vi "Actor.vi"(7 "ConcreteActor":refnum<class "ConcreteActor.lvclass">, 11 "ErrorQueue":refnum<queue>) -> (4 "Error":errorcluster, 5 "ConcreteActor":refnum<class "ConcreteActor.lvclass">)   [LabVIEW 2020, in "_Template.lvlib" / "ActorTemplate.lvlib" / "{{Name}}.lvlib" / "ConcreteActor.lvclass"]
uses:
  ConcreteActor.lvclass
  C:/jettl-harness/repos/jettl/src/jettl/jettl/Actor/Actor.lvclass
  ConcreteActor.lvclass/ConcreteActor.ctl
  jettl/jettl/jettl.lvlib
panel:
  # "This panel can be extended with controls and indicators, though do not modify the conn pane."
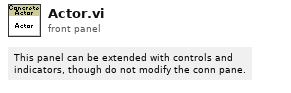
[diagram p1: front panel]
types:
  T1 = cluster{"EventRegistrationRef":refnum<event-registration>}
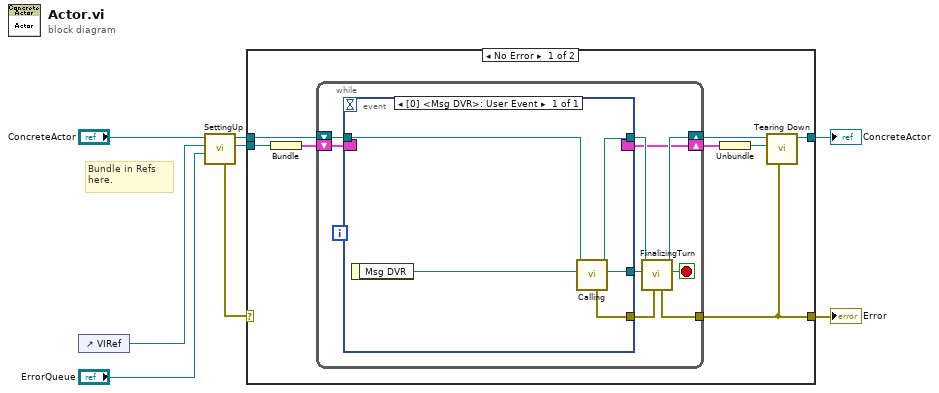
[diagram p0: block diagram]
diagram:
  # "Bundle in Refs here."
  n1 = control-ref of="VIRef"() -> (w3:refnum<vi>)
  n2 = call "SettingUp.vi"("ErrorQueue"="ErrorQueue", "VIRef"=w3, "Actor"="ConcreteActor") -> ("EventRegistrationRef"=w6:refnum<event-registration>, "Actor"=w4:refnum<class "ConcreteActor.lvclass">, "Error"=w1:errorcluster)  [unwired: 6 in]
  n3 = case shown="No Error" w1 {
    selector: w1 -> [_ w31]
    tunnel: [w11 w32] -> w8
    tunnel: w4 -> [w16 w32]
    tunnel: [w10 w31] -> w7
    tunnel: w6 -> [w15 _]
    frame No Error {
      n4 = Bundle("EventRegistrationRef"=w15) -> (w14:T1)  [unwired: 1 in]
      n5 = while {
        shift-right: [w18] -> w12
        shift-left: w16 -> [w25]
        tunnel: [w21] -> w10
        shift-right: [w17] -> w13
        shift-left: w14 -> [w23]
        stop <- w24 stop-if-true
        n6 = event shown="[0] <Msg DVR>: User Event" {
          selector: w23 -> [_]
          dyn-events: [_] -> w17
          timeout: _ -> [_]
          tunnel: w25 -> [w29]
          tunnel: [w28] -> w19
          tunnel: [w27] -> w22
          tunnel: [w26] -> w20
          event User Event {
            n7 = event-data() -> ("Msg DVR"=w30:refnum<data-value>)  [unwired: 1 in]
            n8 = call "Calling.vi"("MessageDVR"=w30, "Actor"=w29) -> ("Message"=w26:refnum<class "Message.lvclass">, "Actor"=w28:refnum<class "ConcreteActor.lvclass">, "Error"=w27:errorcluster)  [unwired: 7 in]
          }
        }
        n9 = call "FinalizingTurn.vi"("Error"=w22, "Message"=w20, "Actor"=w19) -> ("ProceedToTearingDown"=w24:bool, "Actor"=w18:refnum<class "ConcreteActor.lvclass">, "Error"=w21:errorcluster)  [unwired: 6 in]
      }
      n10 = Unbundle(w13) -> ("EventRegistrationRef"=w9:refnum<event-registration>)
      n11 = call "Tearing Down.vi"("Error"=w10, "EventRegistrationRef"=w9, "Actor"=w12) -> ("Actor"=w11:refnum<class "ConcreteActor.lvclass">)  [unwired: 8 in]
    }
    frame Error {
    }
  }
  "ConcreteActor" <- w8
  "Error" <- w7
